vi "7430 Invalid EDS file ident--error.vi"(8 "error in":errorcluster, 11 "Selected EDS File":path) -> (0 "error out":errorcluster)   [LabVIEW 2024, in "UI Actor.lvlib" / "UI Actor.lvclass"]
uses:
  UI Actor.lvclass
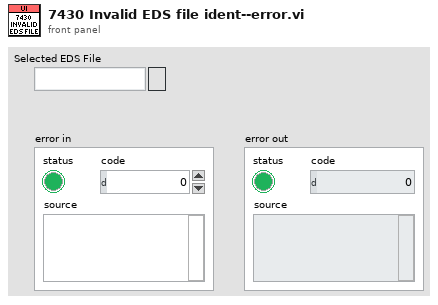
[diagram p1: front panel]
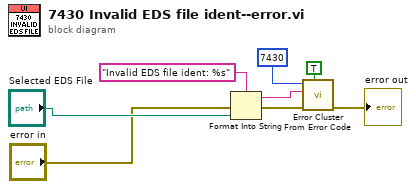
[diagram p0: block diagram]
diagram:
  n1 = Format Into String(format string="Invalid EDS file ident: %s" ("error message (\"\")"), error in="error in", "Selected EDS File") -> (resulting string=w5:string, error out=w4:errorcluster)  [unwired: 1 in]
  n2 = call <vilib>:"Error Cluster From Error Code.vi"("show call chain? (False)"=TRUE, "error in (no error)"=w4, "error message (\"\")"=w5, "error code (0)"=7430) -> ("error out"=→"error out":errorcluster)  [unwired: 5 in]
